vi "setClaseImagen.vi"(8 "error in":errorcluster, 10 "ImageDataIn":T1, 11 "claseImagen in":refnum<class "claseImagen.lvclass">) -> (0 "error out":errorcluster, 3 "claseImagen out":refnum<class "claseImagen.lvclass">)   [LabVIEW 2014, in "claseImagen.lvclass"]
uses:
  claseImagen.lvclass
  claseImagen.lvclass/claseImagen.ctl
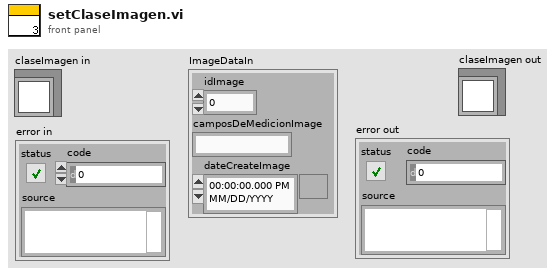
[diagram p1: front panel]
types:
  T1 = cluster{"idImage":dbl, "camposDeMedicionImage":string, "dateCreateImage":timestamp}
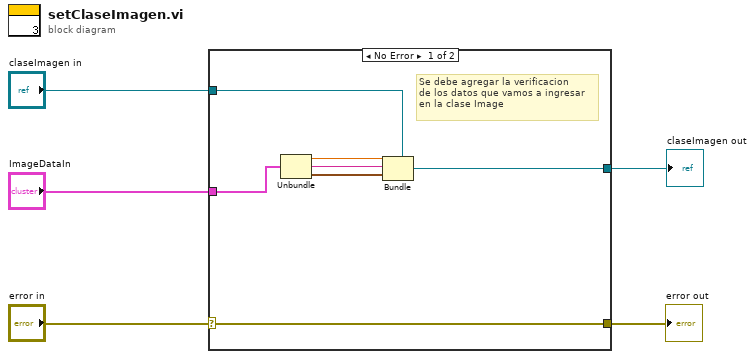
[diagram p0: block diagram]
diagram:
  n1 = case shown="No Error" "error in" {
    selector: "error in" -> [w12 w14]
    tunnel: [w12 w14] -> w4
    tunnel: "claseImagen in" -> [w11 w13]
    tunnel: [w10 w13] -> w2
    tunnel: "ImageDataIn" -> [w9 _]
    frame No Error {
      # "Se debe agregar la verificacion\nde los datos que vamos a ingresar\nen la clase Image"
      n2 = Unbundle(w9) -> ("idImage"=w8:dbl, "camposDeMedicionImage"=w7:string, "dateCreateImage"=w6:timestamp)
      n3 = Bundle(cluster=w11, w8, w7, w6) -> (w10:refnum<class "claseImagen.lvclass">)
    }
    frame Error {
    }
  }
  "claseImagen out" <- w2
  "error out" <- w4
